vi "PlaceChild.vi"(0 "reference in":refnum<class "HGrid.lvclass">, 5 "error in (no error)":errorcluster) -> (14 "reference out":refnum<class "HGrid.lvclass">, 19 "error out":errorcluster)   [LabVIEW 2019, in "HGrid.lvclass"]
uses:
  HGrid.lvclass
  C:/Users/Taylor.Hillegeist/OneDrive - Ultra/LabVIEW/Pgui2/Pgui_Obj_class/Pgui_Obj.lvclass
  Pgui_Obj_class/Pgui_Obj.lvclass
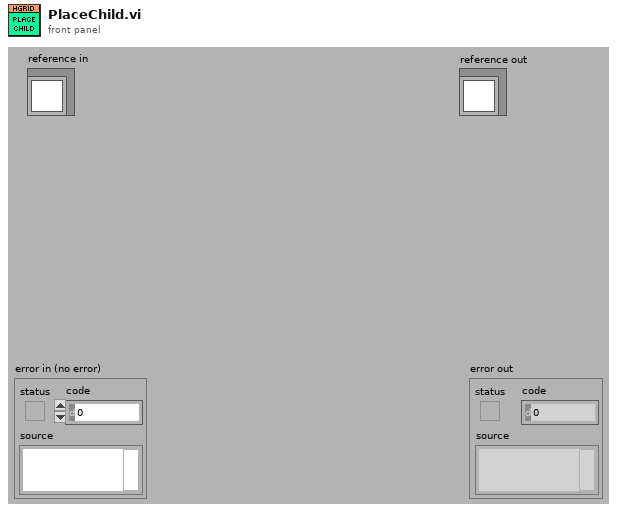
[diagram p1: front panel]
types:
  T1 = cluster{"left":i16, "top":i16, "right":i16, "bottom":i16}
  T2 = typedef "Pgui_Obj.lvclass/ObjectAttributes.ctl" = cluster{"Children":refnum<class "Pgui_Obj.lvclass">[], "Draw Instr":picture, "Params":cluster{"left":i16, "top":i16, "right":i16, "bottom":i16}, "Parent_Pgui_Obj":refnum<class "Pgui_Obj.lvclass">, "MouseOver":bool}
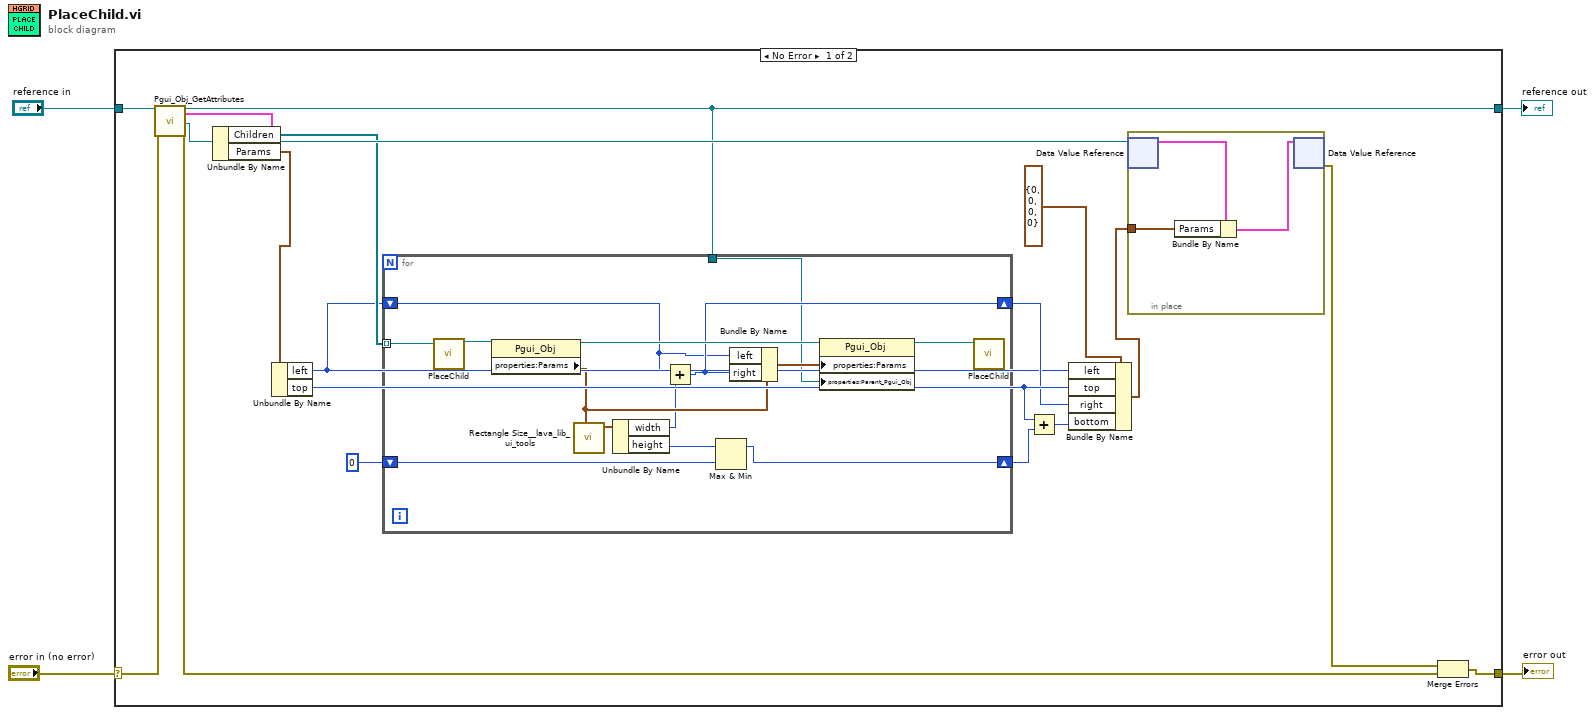
[diagram p0: block diagram]
diagram:
  n1 = case shown="No Error" "error in (no error)" {
    selector: "error in (no error)" -> [w22 w41]
    tunnel: [w19 w41] -> w3
    tunnel: [w6 w40] -> w1
    tunnel: "reference in" -> [w21 w40]
    frame No Error {
      n2 = call "Pgui_Obj_GetAttributes.vi"("reference in"=w21, "error in (no error)"=w22) -> ("reference out"=w6:refnum<class "HGrid.lvclass">, "Data"=w18:T2, "DataRef"=w17:refnum<data-value>, "error out"=w20:errorcluster)  [unwired: 14 in]
      n3 = Unbundle By Name(w18) -> ("Children"=w10:refnum<class "Pgui_Obj.lvclass">[], "Params"=w11:T1)
      n4 = Unbundle By Name(w11) -> ("left"=w5:i16, "top"=w12:i16)
      n5 = for {
        tunnel: w10 -> [w24] mode=indexing
        shift-right: [w34] -> w7
        shift-left: w5 -> [w30]
        shift-right: [w27] -> w13
        shift-left: 0 -> [w29]
        tunnel: w6 -> [w26]
        n6 = call-dynamic "PlaceChild.vi"("reference in"=w24) -> ("reference out"=w23:refnum<class "Pgui_Obj.lvclass">)  [unwired: 17 in, 1 out]
        n7 = property class="Pgui_Obj"(reference=w23) -> (reference out=w36:refnum<class "Pgui_Obj.lvclass">, "properties:Params"=w33:T1)  [unwired: 1 in, 1 out]
        n8 = call <vilib>:"Rectangle Size__lava_lib_ui_tools.vi"("Rectangle"=w33) -> ("Rect Size"=w32:cluster{"width":i32, "height":i32})  [unwired: 8 in, 2 out]
        n9 = Unbundle By Name(w32) -> ("width"=w31:i32, "height"=w28:i32)
        n10 = Add(x=w30, y=w31) -> (x+y=w34:i32)
        n11 = Max & Min(x=w28, y=w29) -> (max(x,y)=w27:i32)  [unwired: 1 out]
        n12 = Bundle By Name(cluster=w33, "left"=w30, "right"=w34) -> (w35:T1)
        n13 = property class="Pgui_Obj"(reference=w36, "properties:Params"=w35, "properties:Parent_Pgui_Obj"=w26) -> (reference out=w25:refnum<class "Pgui_Obj.lvclass">)  [unwired: 1 in, 1 out]
        n14 = call-dynamic "PlaceChild.vi"("reference in"=w25) -> ()  [unwired: 17 in, 2 out]
      }
      n15 = Add(x=w12, y=w13) -> (x+y=w14:i32)
      n16 = Bundle By Name(cluster=T1 {"left"=0, "top"=0, "right"=0, "bottom"=0} ("Rectangle"), "left"=w5, "top"=w12, "right"=w7, "bottom"=w14) -> (w8:T1)
      n17 = in-place {
        in-place-border: w8 -> [w37]
        n18 = in-place-dvr #1(w17) -> (w39:T2)  [unwired: 1 out]
        n19 = Bundle By Name(cluster=w39, "Params"=w37) -> (w38:T2)
        n20 = in-place-dvr #1(w38) -> (w16:errorcluster)  [unwired: 1 out]
      }
      n21 = Merge Errors(w16, w20) -> (w19:errorcluster)
    }
    frame Error {
    }
  }
  "error out" <- w3
  "reference out" <- w1
